vi "Set G08 Trigger Parameters.vi"(7 "DG Number":i32, 8 "error in (no error)":errorcluster, 11 "Settings":T1={"Gate Terminate"=TRUE, "Gate Level"=1.0, "Gate Delay (µs)"=0.0, "Gate Type"=TRUE, "Synchronize Gate"=FALSE, "Force Trigger (µs)"=0.0, "Step Back Time (µs)"=0.0, "Burst Counter"=0, "MS Bus"=8} {"MS Bus" format="%04x" items=["Local Primary"=1, "Local Secondary"=2, "Local Force"=4, "Resynchronize"=8, "Master Primary"=16, "Master Secondary"=32, "Master Force"=64, "System Clock"=128, "Delay Clock"=256, "Inhibit Local"=512, "Start Local"=1024, "Start Bus"=2048, "Step Back Local"=4096, "Step Back Bus"=8192, "From E"=65536, "From F"=131072, "From Bus"=262144]; "Step Back Time (µs)" min=0.0 format="%.6f"; "Force Trigger (µs)" min=0.0 format="%.6f"; "Gate Delay (µs)" format="%.3f"; "Gate Level" min=-2.5 max=2.5 format="%.3g"}) -> (0 "error out":errorcluster)   [LabVIEW 2009]
doc: "long Set_TriggerParameters(BOOL TriggerTerminate, double InternalClock, double TriggerLevel, unsigned long PresetValue, unsigned long GateDivider, BOOL PositiveGate, BOOL InternalTrigger, BOOL InternalArm, BOOL SoftwareTrigger, BOOL RisingEdge, BOOL StopOnPreset, BOOL ResetWhenDone, BOOL TriggerEnable, long DG_Number);"
uses:
  BME DLL/DelayGenerator.dll
panel:
  # "NOTICE -- YOU MUST LEAVE THIS NOTICE IN PLACE.  PER THE TERMS OF THE LICENSE BELOW, YOU MAY SUBLICENSE THIS SOFTWARE \nIN ANY WAY THAT DOES NOT CONFLICT WITH THIS LICENSE.\n\n### BSD License (http://www.opensource.org/licenses/bsd-license.php) Begin ###\n \nCopyright (c) 2011, Applied Energetics, http://www.appliedenergetics.com,\n                               Richard Schwerdtfeger, <rschwerdtfeger@appliedenergetics.com>\n\nAll rights reserved.\n\nRedistribution and use in source and binary forms, with or without modification, are permitted provided that the \nfollowing conditions are met:\n\n    * Redistributions of source code must retain the above copyright notice, this list of conditions and the following disclaimer.\n    * Redistributions in binary form must reproduce the above copyright notice, this list of conditions and the following disclaimer \n       in the documentation and/or other materials provided with the distribution.\n    * Neither the name of Richard Schwerdtfeger, Applied Energetics, Inc., nor the names of its contributors may be used to \n       endorse or promote products derived from this software without specific prior written permission.\n\nTHIS SOFTWARE IS PROVIDED BY THE COPYRIGHT HOLDERS AND CONTRIBUTORS \"AS IS\" AND ANY EXPRESS OR IMPLIED WARRANTIES, \nINCLUDING, BUT NOT LIMITED TO, THE IMPLIED WARRANTIES OF MERCHANTABILITY AND FITNESS FOR A PARTICULAR PURPOSE ARE \nDISCLAIMED. IN NO EVENT SHALL THE COPYRIGHT OWNER OR CONTRIBUTORS BE LIABLE FOR ANY DIRECT, INDIRECT, INCIDENTAL,\n SPECIAL, EXEMPLARY, OR CONSEQUENTIAL DAMAGES (INCLUDING, BUT NOT LIMITED TO, PROCUREMENT OF SUBSTITUTE GOODS OR \nSERVICES; LOSS OF USE, DATA, OR PROFITS; OR BUSINESS INTERRUPTION) HOWEVER CAUSED AND ON ANY THEORY OF LIABILITY, \nWHETHER IN CONTRACT, STRICT LIABILITY, OR TORT (INCLUDING NEGLIGENCE OR OTHERWISE) ARISING IN ANY WAY OUT OF THE USE \nOF THIS SOFTWARE, EVEN IF ADVISED OF THE POSSIBILITY OF SUCH DAMAGE.\n\n### BSD License End ###"
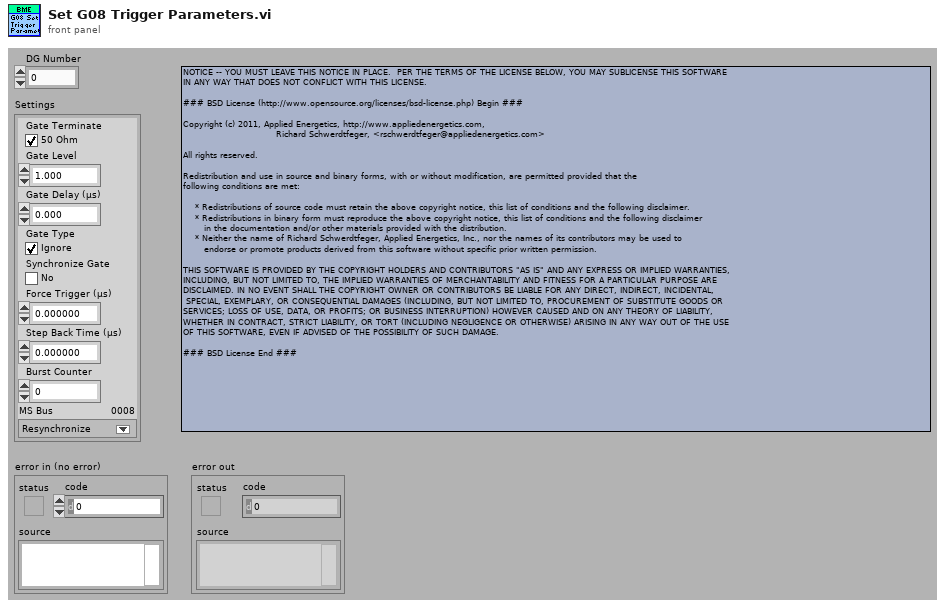
[diagram p1: front panel]
types:
  T1 = cluster{"Gate Terminate":bool, "Gate Level":dbl, "Gate Delay (µs)":dbl, "Gate Type":bool, "Synchronize Gate":bool, "Force Trigger (µs)":dbl, "Step Back Time (µs)":dbl, "Burst Counter":u32, "MS Bus":u32}
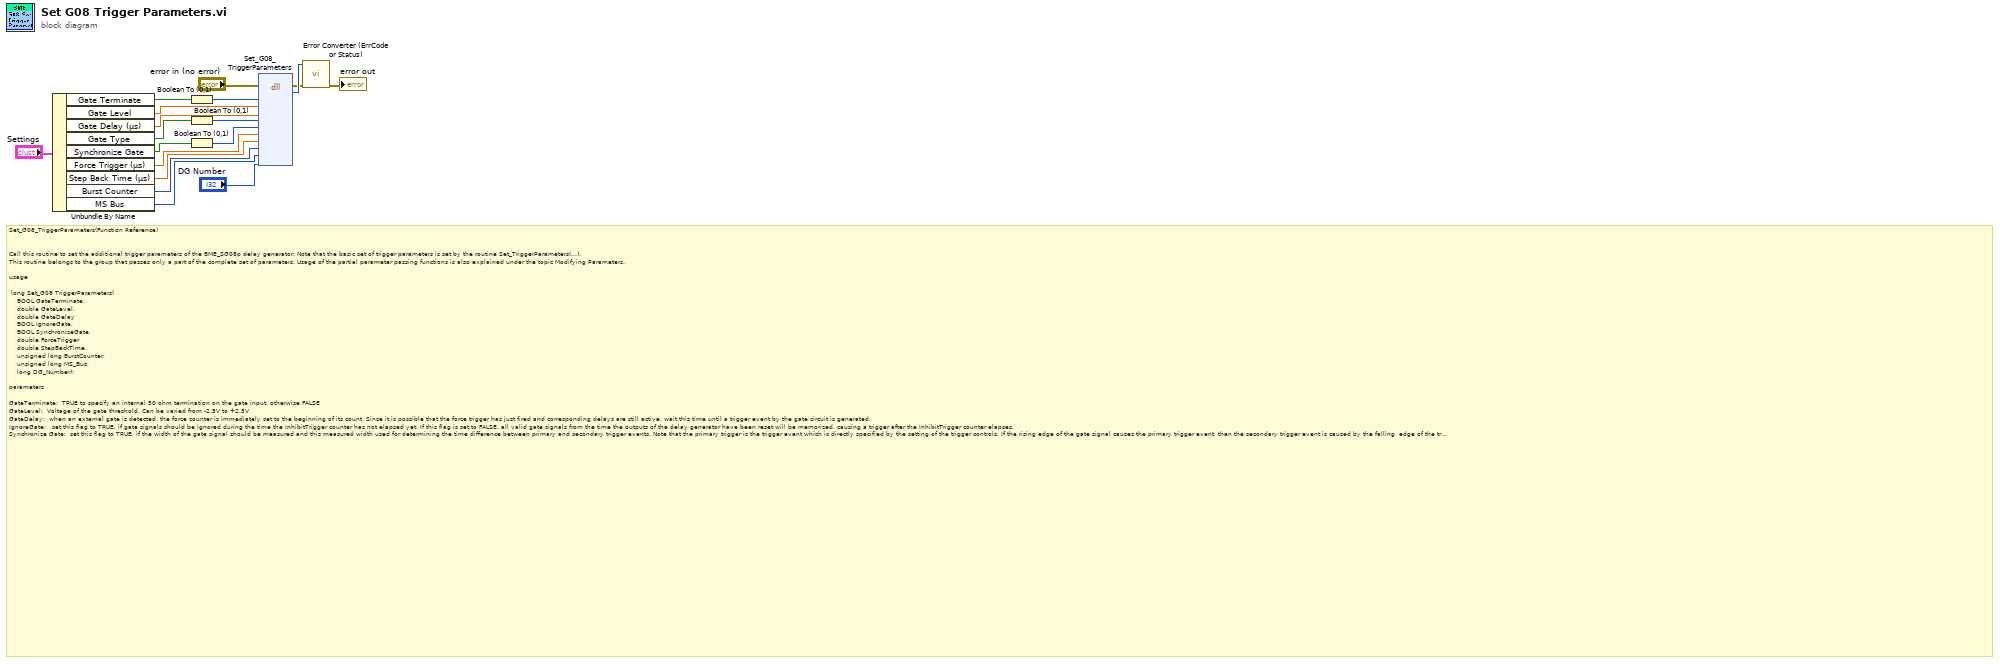
[diagram p0: block diagram]
diagram:
  # "Set_G08_TriggerParameters(Function Reference)\n\n\nCall this routine to set the additional trigger parameters of the BME_SG08p delay generator. Note that the basic set of trigger parameters is set by the routine Set_TriggerParameters(...).\nThis routine belongs to the group that passes only a part of the complete set of parameters. Usage of the partial parameter passing functions is also explained under the topic Modifying Parameters.\n\nusage\n\n\tlong Set_G08 TriggerParameters(\n\t\t\t\tBOOL GateTerminate, \n\t\t\t\tdouble GateLevel,\n\t\t\t\tdouble GateDelay\n\t\t\t\tBOOL IgnoreGate, \n\t\t\t\tBOOL SynchronizeGate, \n\t\t\t\tdouble ForceTrigger\n\t\t\t\tdouble StepBackTime, \n\t\t\t\tunsigned long BurstCounter,\n\t\t\t\tunsigned long MS_Bus, \n\t\t\t\tlong DG_Number);\n\nparameters\n\nGateTerminate:\t\tTRUE to specify an internal 50 ohm termination on the gate input, otherwise FALSE\nGateLevel:\t\tVoltage of the gate threshold. Can be varied from -2.5V to +2.5V\nGateDelay:\t\twhen an external gate is detected, the force counter is immediately set to the beginning of its count. Since it is possible that the force trigger has just fired and corresponding delays are still active, wait this time until a trigger event by the gate circuit is generated. \nIgnoreGate: \t\tset this flag to TRUE, if gate signals should be ignored during the time the InhibitTrigger counter has not elapsed yet. If this flag is set to FALSE, all valid gate signals from the time the outputs of the delay generator have been reset will be memorized, causing a trigger after the InhibitTrigger counter elapses.\nSynchronize Gate: \tset this flag to TRUE, if the width of the gate signal should be measured and this measured width used for determining the time difference between primary and secondary trigger events. Note that the primary trigger is the trigger event which is directly specified by the setting of the trigger controls. If the rising edge of the gate signal causes the primary trigger event, then the secondary trigger event is caused by the falling  edge of the trigger signal.\nForceTrigger:\t\ttime in µsec after a valid trigger event, that the delay generator will be triggered again internally.\nStepBackTime:\t\ttime in µsec after a valid trigger event, that the delay lists will be stepped back according to the value pointed to by the step back array.\nBurstCounter:\t\tentering a nonzero number into this control will generate a corresponding number of triggers after a valid external trigger event. The time difference between trigger events of this burst is defined by the inhibit time.\nMS_Bus:\t\tonly one bit of this unsigned long parameter is used: (The corresponding constants are defined in ‘’DG_Data.h’’.)\n   Resynchronize = 0x8: \t\tif the clock signal placed on the master/salve bus is prescaled, i.e. of lower frequency than the input clock signal, the clock signal on the master/slave bus is resynchronized to the nearest clock period of the input clock signal.\nDG_Number:\t\tThe number of the delay generator as assigned by the Initialize_DG_BME routine\n\nreturn value\n\n\t0:  success\n\t2:  DG_Number is out of range"
  n1 = Unbundle By Name("Settings") -> ("Gate Terminate"=w6:bool, "Gate Level"=w9:dbl, "Gate Delay (µs)"=w8:dbl, "Gate Type"=w4:bool, "Synchronize Gate"=w3:bool, "Force Trigger (µs)"=w7:dbl, "Step Back Time (µs)"=w10:dbl, "Burst Counter"=w11:u32, "MS Bus"=w12:u32)
  n2 = Boolean To (0,1)(Boolean=w6) -> (0, 1=w5:i16)
  n3 = Boolean To (0,1)(Boolean=w4) -> (0, 1=w1:i16)
  n4 = Boolean To (0,1)(Boolean=w3) -> (0, 1=w2:i16)
  n5 = dll-call lib="C:/Dokumente und Einstellungen/A2.5/Desktop/POLARIS BME DG/BME DLL/DelayGenerator.dll" fn="Set_G08_TriggerParameters"(error in="error in (no error)", "GateTerminate"=w5, "GateLevel"=w9, "GateDelay"=w8, "IgnoreGate"=w1, "SynchronizeGate"=w2, "ForceTrigger"=w7, "StepBackTime"=w10, "BurstCounter"=w11, "MS_Bus"=w12, "DG_Number"="DG Number") -> (error out=w16:errorcluster, "return type"=w18:i32)  [unwired: 12 in, 1 out]
  n6 = call "Error Converter (ErrCode or Status).vi"("error in (no error)"=w16, "error code"=w18) -> ("error out"=→"error out":errorcluster)  [unwired: 9 out]
